vi "Initialize.vi"(8 "error in":errorcluster, 11 "GMW in":refnum<class "GMW.lvclass">) -> (0 "error out":errorcluster, 3 "GMW out":refnum<class "GMW.lvclass">)   [LabVIEW 2015, in "GMW.lvclass"]
uses:
  GMW.lvclass
  DMA.lvclass/DMA.ctl
  Accessors/Write ri.vi
  Accessors/Write ro.vi
  Accessors/Write Leff.vi
  DMA.lvclass
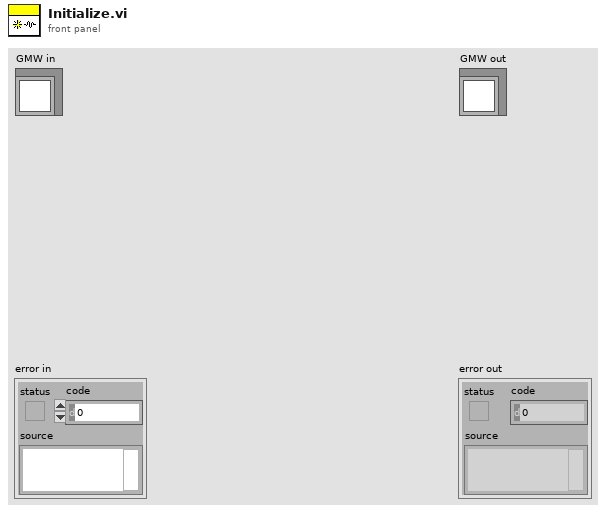
[diagram p1: front panel]
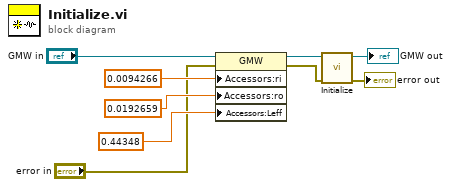
[diagram p0: block diagram]
diagram:
  n1 = property class="GMW"(reference="GMW in", error in="error in", "Accessors:ri"=0.0094266 ("ri"), "Accessors:ro"=0.0192659 ("ro"), "Accessors:Leff"=0.44348 ("Leff")) -> (reference out=w9:refnum<class "GMW.lvclass">, error out=w5:errorcluster)
  n2 = call-parent "Initialize.vi"("error in"=w5, "DMA in"=w9) -> ("error out"=→"error out":errorcluster, "DMA out"=→"GMW out":refnum<class "GMW.lvclass">)  [unwired: 8 in]
